vi "sv_Get SV Property Name String.vi"(7 "property":T1 items=["Engineering units", "Custom unit label", "Weighting filter", "Pregain", "Octave standard", "Octave bandwidth", "Octave low band", "Octave high band", "Spectrum skewed", "Samples / revolution", "Order", "Tachometer", "Pulses Per Revolution", "Rotation Direction", "Probe Angle", "Pair", "Channel Alias", "Tachometer Threshold", "Tachometer Slope", "Max Order", "Sensor Location", "Sensor Orientation", "Analog Software Trigger", "Trigger Level", "Pretrigger Samples", "Trigger Slope", "Trigger Hysteresis", "Sensor sensitivity", "Sensor type", "Sensor maximum", "Complimentary Spectrum Type"]) -> (6 "TDMS property name":string, 10 "WDT attribute name":string)   [LabVIEW 2017]
uses:
  <vilib>/addons/_NISVFA/_Shared subVIs/Controls/SV Channel Properties.ctl
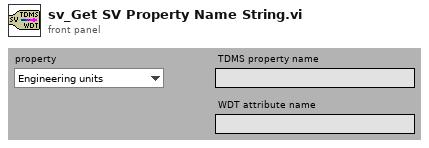
[diagram p1: front panel]
types:
  T1 = typedef "SV Channel Properties.ctl" = u16
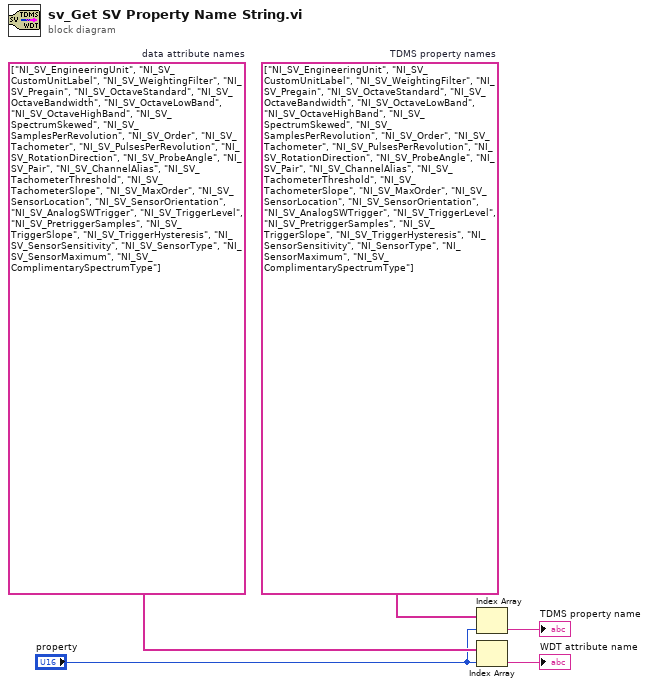
[diagram p0: block diagram]
diagram:
  w3 = string[] ["NI_SV_EngineeringUnit", "NI_SV_CustomUnitLabel", "NI_SV_WeightingFilter", "NI_SV_Pregain", "NI_SV_OctaveStandard", "NI_SV_OctaveBandwidth", "NI_SV_OctaveLowBand", "NI_SV_OctaveHighBand", "NI_SV_SpectrumSkewed", "NI_SV_SamplesPerRevolution", "NI_SV_Order", "NI_SV_Tachometer", "NI_SV_PulsesPerRevolution", "NI_SV_RotationDirection", "NI_SV_ProbeAngle", "NI_SV_Pair", "NI_SV_ChannelAlias", "NI_SV_TachometerThreshold", "NI_SV_TachometerSlope", "NI_SV_MaxOrder", "NI_SV_SensorLocation", "NI_SV_SensorOrientation", "NI_SV_AnalogSWTrigger", "NI_SV_TriggerLevel", "NI_SV_PretriggerSamples", "NI_SV_TriggerSlope", "NI_SV_TriggerHysteresis", "NI_SensorSensitivity", "NI_SensorType", "NI_SensorMaximum", "NI_SV_ComplimentarySpectrumType"]  # TDMS property names
  w5 = string[] ["NI_SV_EngineeringUnit", "NI_SV_CustomUnitLabel", "NI_SV_WeightingFilter", "NI_SV_Pregain", "NI_SV_OctaveStandard", "NI_SV_OctaveBandwidth", "NI_SV_OctaveLowBand", "NI_SV_OctaveHighBand", "NI_SV_SpectrumSkewed", "NI_SV_SamplesPerRevolution", "NI_SV_Order", "NI_SV_Tachometer", "NI_SV_PulsesPerRevolution", "NI_SV_RotationDirection", "NI_SV_ProbeAngle", "NI_SV_Pair", "NI_SV_ChannelAlias", "NI_SV_TachometerThreshold", "NI_SV_TachometerSlope", "NI_SV_MaxOrder", "NI_SV_SensorLocation", "NI_SV_SensorOrientation", "NI_SV_AnalogSWTrigger", "NI_SV_TriggerLevel", "NI_SV_PretriggerSamples", "NI_SV_TriggerSlope", "NI_SV_TriggerHysteresis", "NI_SV_SensorSensitivity", "NI_SV_SensorType", "NI_SV_SensorMaximum", "NI_SV_ComplimentarySpectrumType"]  # data attribute names
  n1 = Index Array(array=w3, index="property") -> (element=→"TDMS property name":string)
  n2 = Index Array(array=w5, index="property") -> (element=→"WDT attribute name":string)
